vi "DDFL_Controller_v11mai.vi"(0 "K":dbl[](array[numeric]), 1 "q_ref":dbl[](array[numeric]), 2 "q1":dbl, 3 "q2":dbl, 4 "q3":dbl, 5 "q4":dbl) -> (16 "u_out":dbl)   [LabVIEW 2021]
uses:
  <vilib>/Analysis/baseanly.llb/Real A x B.vi
  <vilib>/Analysis/Matrix/Numeric/Conversions/Matrix To Array - RM.vi
  <vilib>/Analysis/Matrix/Numeric/Conversions/Array To Matrix - RA2.vi
  <vilib>/Analysis/Matrix/NI_Matrix.lvlib
  <vilib>/Analysis/NI_AALBase.lvlib
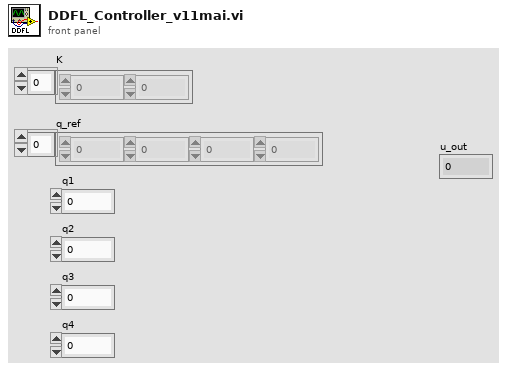
[diagram p1: front panel]
types:
  T1 = typedef "NI_Matrix.lvlib/RealMatrix.ctl" = dbl[][]
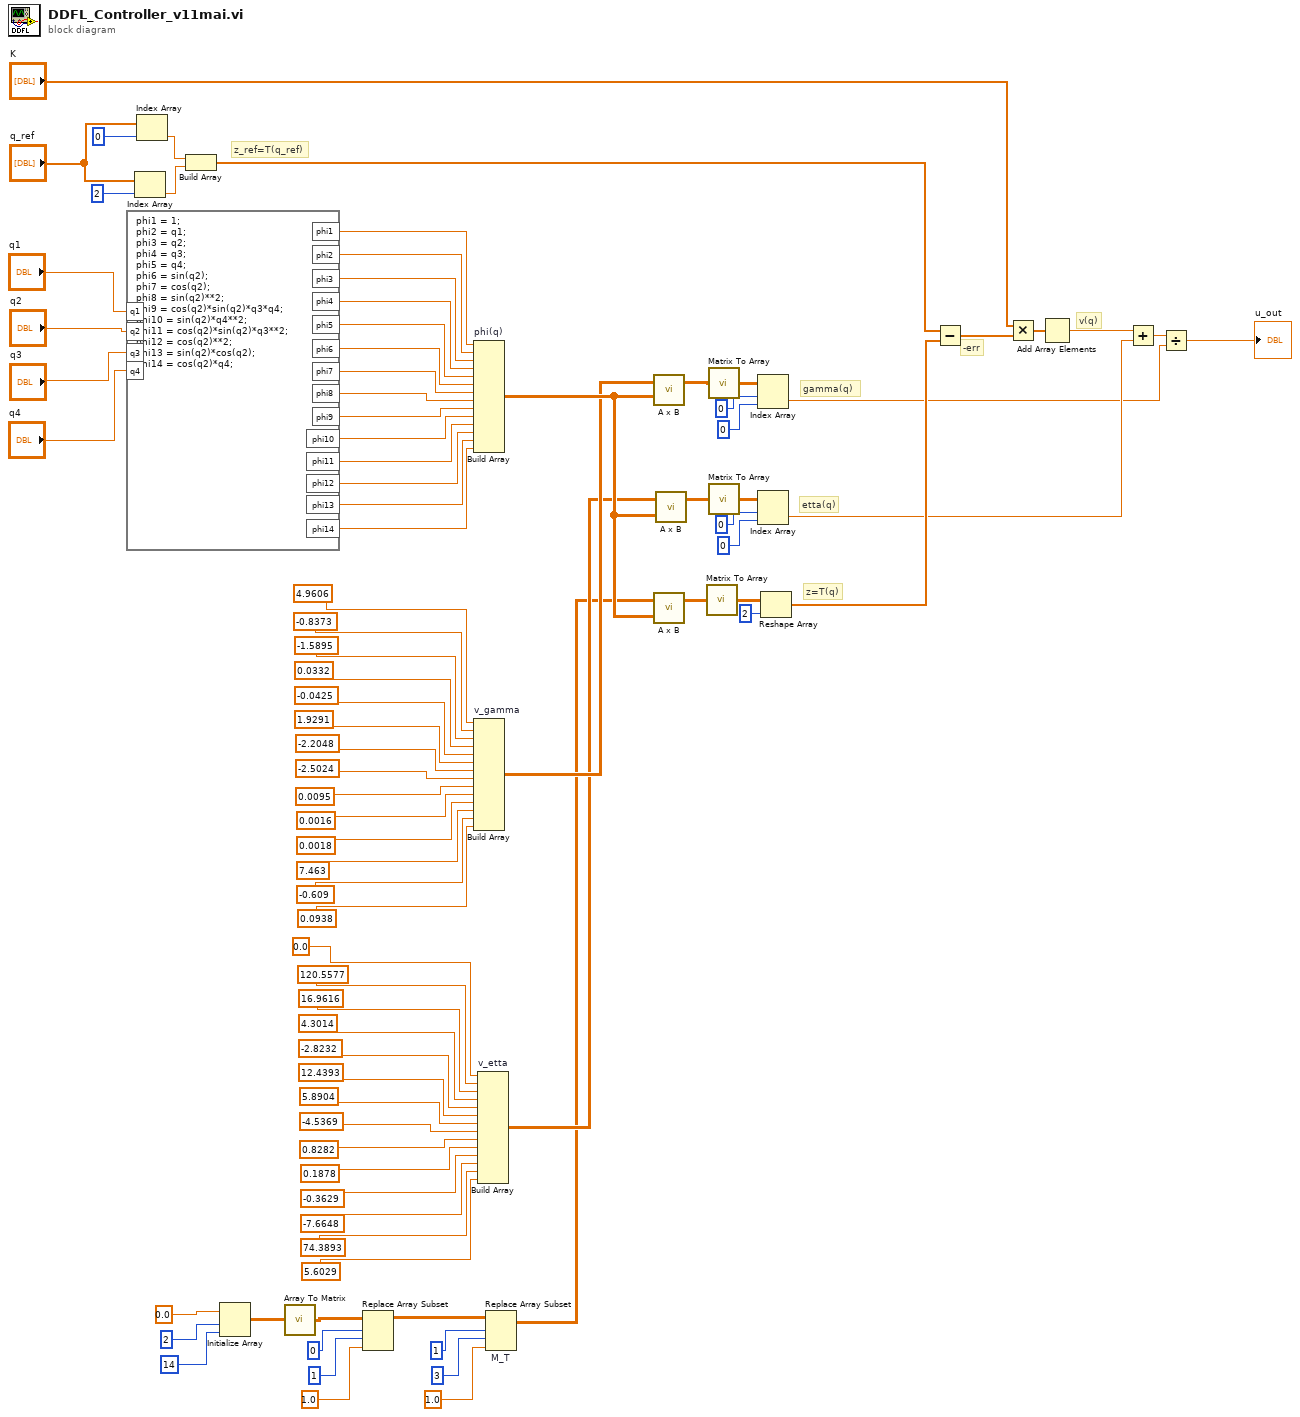
[diagram p0: block diagram]
diagram:
  # "v(q)"
  # "-err"
  # "z_ref=T(q_ref)"
  # "z=T(q)"
  # "etta(q)"
  # "gamma(q)"
  n1 = formula code="phi1 = 1;\nphi2 = q1;\nphi3 = q2;\nphi4 = q3;\nphi5 = q4;\nphi6 = sin(q2);\nphi7 = cos(q2);\nphi8 = sin(q2)**2;\nphi9 = cos(q2)*sin(q2)*q3*q4;\nphi10 = sin(q2)*q4**2;\nphi11 = cos(q2)*sin(q2)*q3**2;\nphi12 = cos(q2)**2;\nphi13 = sin(q2)*cos(q2);\nphi14 = cos(q2)*q4;"("q1"="q1", "q2"="q2", "q3"="q3", "q4"="q4") -> ("phi1"=w88:dbl, "phi2"=w87:dbl, "phi3"=w86:dbl, "phi4"=w85:dbl, "phi5"=w84:dbl, "phi6"=w83:dbl, "phi7"=w82:dbl, "phi8"=w81:dbl, "phi9"=w80:dbl, "phi10"=w79:dbl, "phi11"=w78:dbl, "phi12"=w77:dbl, "phi13"=w76:dbl, "phi14"=w75:dbl)
  n2 = Index Array(array="q_ref", index=2 ("index 3")) -> (element=w13:dbl)
  n3 = Index Array(array="q_ref", index=0 ("index 3")) -> (element=w14:dbl)
  n4 = Build Array(w14, w13) -> (w9:dbl[])
  n5 = Initialize Array(0.0, 2, 14) -> (w43:dbl[][])
  n6 = call-poly <vilib>:"Array To Matrix.vi"("Real 2D Array"=w43) -> ("Real Matrix"=w42:T1)
  n7 = Replace Array Subset(array=w42, new element=1.0, index (row)=0, index (col)=1) -> (w35:T1)
  n8 = Build Array "phi(q)"(w88, w87, w86, w85, w84, w83, w82, w81, w80, w79, w78, w77, w76, w75) -> (w34:T1)
  n9 = Build Array "v_gamma"(4.9606, -0.8373, -1.5895, 0.0332, -0.0425, 1.9291, -2.2048, -2.5024, 0.0095, 0.0016, 0.0018, 7.463, -0.609, 0.0938) -> (w33:T1)
  n10 = Build Array "v_etta"(0.0, 120.5577, 16.9616, 4.3014, -2.8232, 12.4393, 5.8904, -4.5369, 0.8282, 0.1878, -0.3629, -7.6648, 74.3893, 5.6029) -> (w32:T1)
  n11 = Replace Array Subset "M_T"(array=w35, new element=1.0, index (row)=1, index (col)=3) -> (w31:T1)
  n12 = call-poly <vilib>:"A x B.vi"("B"=w34, "A"=w33) -> ("A x B"=w23:T1)  [unwired: 1 out]
  n13 = call-poly <vilib>:"A x B.vi"("B"=w34, "A"=w31) -> ("A x B"=w19:T1)  [unwired: 1 out]
  n14 = call-poly <vilib>:"A x B.vi"("B"=w34, "A"=w32) -> ("A x B"=w18:T1)  [unwired: 1 out]
  n15 = call-poly <vilib>:"Matrix To Array.vi"("Real Matrix"=w19) -> ("Real 2D Array"=w12:dbl[][])
  n16 = call-poly <vilib>:"Matrix To Array.vi"("Real Matrix"=w23) -> ("Real 2D Array"=w26:dbl[][])
  n17 = call-poly <vilib>:"Matrix To Array.vi"("Real Matrix"=w18) -> ("Real 2D Array"=w22:dbl[][])
  n18 = Index Array ("Index Array 2")(array=w26, index (row)=0 ("index 3"), index (col)=0 ("index 4")) -> (element=w4:dbl)
  n19 = Index Array ("Index Array 2")(array=w22, index (row)=0 ("index 3"), index (col)=0 ("index 4")) -> (element=w6:dbl)
  n20 = Reshape Array(w12, 2 ("dimension size")) -> (w10:dbl[])
  n21 = Subtract(x=w9, y=w10) -> (x-y=w7:dbl[])
  n22 = Multiply(x="K", y=w7) -> (x*y=w2:dbl[])
  n23 = Add Array Elements(numeric array=w2) -> (sum=w1:dbl)
  n24 = Add(x=w1, y=w6) -> (x+y=w5:dbl)
  n25 = Divide(x=w5, y=w4) -> (x/y=→"u_out":dbl)
